vi "Q_Get Type distances for Athlete individual.vi"(8 "error in (no error)":errorcluster, 10 "Alias":string, 11 "Data Manager in":refnum<class "Data Manager.lvclass">) -> (0 "error out":errorcluster, 1 "Array":dbl[](array[numeric]), 2 "output cluster":cluster{dbl, dbl, dbl}, 3 "Data Manager out":refnum<class "Data Manager.lvclass">)   [LabVIEW 2020, in "Data Manager.lvclass"]
uses:
  Data Manager.lvclass
  Data Manager.lvclass/Data Manager.ctl
  <vilib>/drjdpowell/SQLite Library/SQL Connection/Execute SQL (Single DBL).vi
  <vilib>/drjdpowell/SQLite Library/SQLite.lvlib
  <vilib>/drjdpowell/SQLite Library/SQL Connection/Connection.lvclass
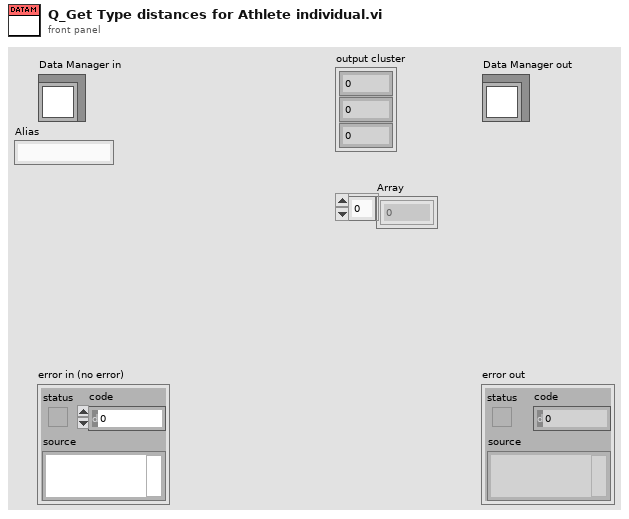
[diagram p1: front panel]
types:
  T1 = cluster{"Result":dbl, "Result":dbl, "Result":dbl}
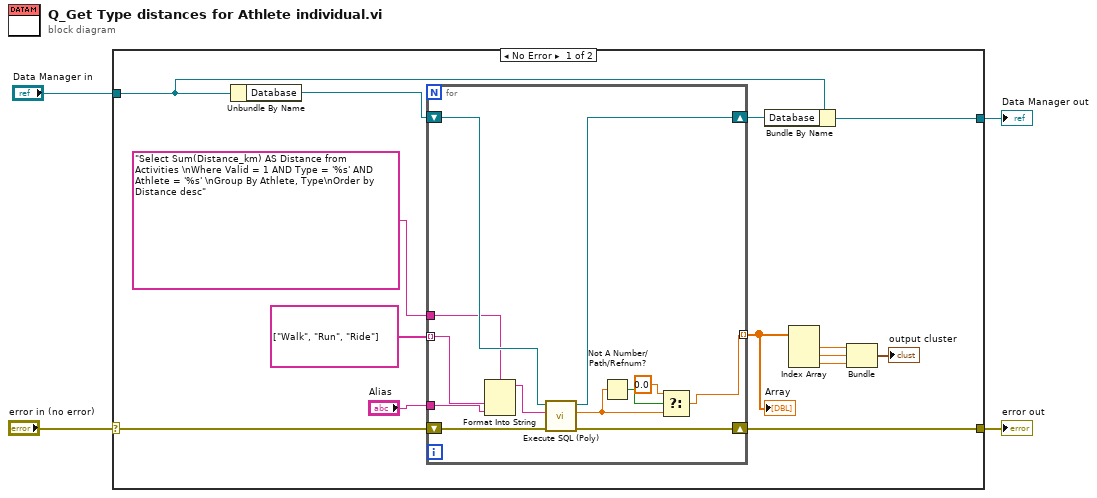
[diagram p0: block diagram]
diagram:
  n1 = case shown="No Error" "error in (no error)" {
    selector: "error in (no error)" -> [w14 w32]
    tunnel: [w13 w32] -> w3
    tunnel: [w16 w31] -> w1
    tunnel: "Data Manager in" -> [w17 w31]
    frame No Error {
      n2 = Unbundle By Name(w17) -> ("Database"=w18:refnum<class "Connection.lvclass">)
      n3 = for {
        tunnel: "Select Sum(Distance_km) AS Distance from Activities \nWhere Valid = 1 AND Type = '%s' AND Athlete = '%s' \nGroup By Athlete, Type\nOrder by Distance desc" ("SQL") -> [w26]
        shift-right: [w29] -> w15
        shift-left: w18 -> [w30]
        shift-right: [w27] -> w13
        shift-left: w14 -> [w28]
        tunnel: string[] ["Walk", "Run", "Ride"] -> [w24] mode=indexing
        tunnel: "Alias" -> [w23]
        tunnel: [w19] -> w9 mode=indexing
        n4 = Format Into String(format string=w26, w24, w23) -> (resulting string=w25:string)  [unwired: 2 in, 1 out]
        n5 = call-poly <vilib>:"Execute SQL (Poly).vi"("error in (no error)"=w28, "SQL"=w25, "SQLite Connection in"=w30) -> ("error out"=w27:errorcluster, "Result"=w20:dbl, "SQLite Connection"=w29:refnum<class "Connection.lvclass">)  [unwired: 6 in]
        n6 = Not A Number/Path/Refnum?(number/path/refnum=w20) -> (NaN/Path/Refnum?=w22:bool)
        n7 = Select(t=0.0, s=w22, f=w20) -> (s? t:f=w19:dbl)
      }
      "Array" <- w9
      n8 = Bundle By Name(cluster=w17, "Database"=w15) -> (w16:refnum<class "Data Manager.lvclass">)
      n9 = Index Array(array=w9) -> (element #1=w7:dbl, element #2=w5:dbl, element #3=w6:dbl)  [unwired: 3 in]
      n10 = Bundle("Result"=w7, "Result"=w5, "Result"=w6) -> (→"output cluster":T1)  [unwired: 1 in]
    }
    frame Error {
    }
  }
  "error out" <- w3
  "Data Manager out" <- w1
